vi "设置styles.vi"(8 "错误输入（无错误）":errorcluster, 9 "外观属性":T1={"大小"=20, "粗体"=FALSE, "下划线"=FALSE, "斜体"=FALSE, "背景色"=16448250, "前景色"=16716509, "Font"=""}, 10 "设置项":i32(ring) items=["Default"=32, "LineNumber"=33, "BraceLight"=34, "BraceBad"=35, "IndentGuide"=37, "CallTip"=38, "FoldDisaplayText"=39], 11 "Scintilla":refnum<k24>) -> (0 "错误输出":errorcluster, 3 "Scintilla":refnum<k24>)   [LabVIEW 2018]
uses:
  ScintillaNET.dll
  System.Drawing
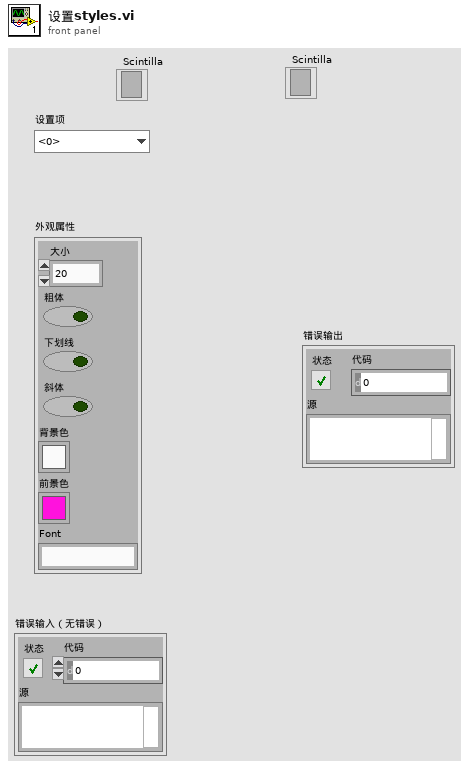
[diagram p1: front panel]
types:
  T1 = cluster{"大小":i32, "粗体":bool, "下划线":bool, "斜体":bool, "背景色":u32, "前景色":u32, "Font":string}
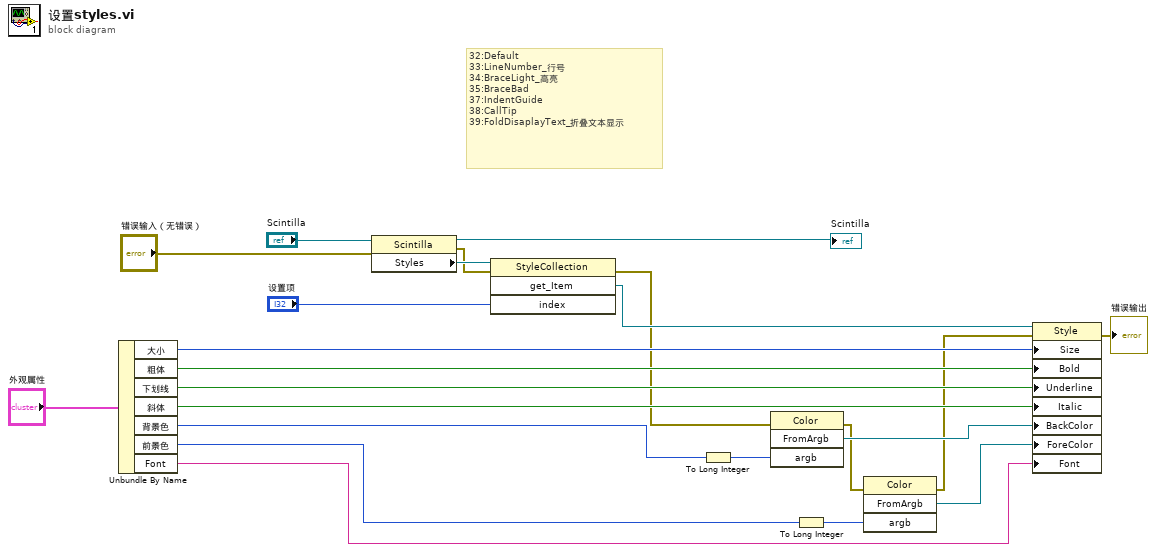
[diagram p0: block diagram]
diagram:
  # "32:Default\n33:LineNumber_行号\n34:BraceLight_高亮\n35:BraceBad\n37:IndentGuide\n38:CallTip\n39:FoldDisaplayText_折叠文本显示"
  n1 = Unbundle By Name("外观属性") -> ("大小"=w13:i32, "粗体"=w12:bool, "下划线"=w11:bool, "斜体"=w10:bool, "背景色"=w9:u32, "前景色"=w8:u32, "Font"=w1:string)
  n2 = property class="Scintilla"(reference="Scintilla", error in="错误输入（无错误）") -> (reference out=→"Scintilla":refnum<k24>, error out=w6:errorcluster, "Styles"=w23:refnum<k24>)
  n3 = invoke class="StyleCollection" method="get_Item"(reference=w23, error in=w6, "index"="设置项") -> (error out=w5:errorcluster, "get_Item"=w22:refnum<k24>)  [unwired: 1 in, 2 out]
  n4 = To Long Integer(number=w9) -> (32bit integer=w21:i32)
  n5 = invoke class="Color" method="FromArgb"(error in=w5, "argb"=w21) -> (error out=w4:errorcluster, "FromArgb"=w18:refnum<k24>)  [unwired: 2 in, 2 out]
  n6 = To Long Integer(number=w8) -> (32bit integer=w20:i32)
  n7 = invoke class="Color" method="FromArgb"(error in=w4, "argb"=w20) -> (error out=w3:errorcluster, "FromArgb"=w19:refnum<k24>)  [unwired: 2 in, 2 out]
  n8 = property class="Style"(reference=w22, error in=w3, "Size"=w13, "Bold"=w12, "Underline"=w11, "Italic"=w10, "BackColor"=w18, "ForeColor"=w19, "Font"=w1) -> (error out=→"错误输出":errorcluster)  [unwired: 1 out]
